vi "Theta_AxisMotorControlSetupAndHome.vi"(11 "Automation Refnum in":refnum<k7>(container)) -> (2 "Angle Serial Number":i32=40808764, 3 "Automation Refnum out":refnum<k7>)   [LabVIEW 2020]
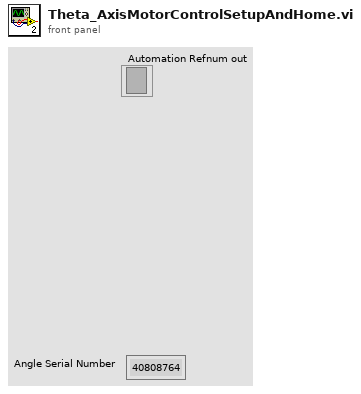
[diagram p1: front panel]
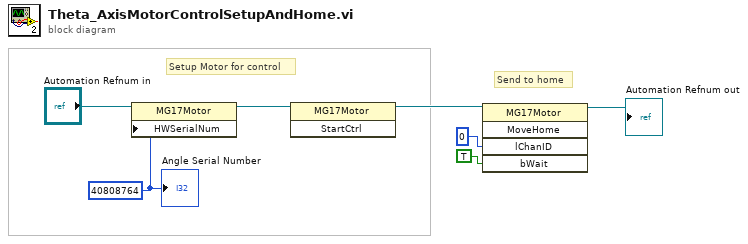
[diagram p0: block diagram]
diagram:
  w6 = 40808764 ("Serial Number Number")
  # "Setup Motor for control"
  # "Send to home"
  n1 = property on="Property Node" class="MG17Motor"(reference="Automation Refnum in", "HWSerialNum"=w6) -> (reference out=w2:refnum<k7>)  [unwired: 1 in, 1 out]
  n2 = invoke class="MG17Motor" method="StartCtrl"(reference=w2) -> (reference out=w1:refnum<k7>)  [unwired: 2 in, 2 out]
  n3 = invoke class="MG17Motor" method="MoveHome"(reference=w1, "lChanID"=0, "bWait"=TRUE) -> (reference out=→"Automation Refnum out":refnum<k7>)  [unwired: 2 in, 4 out]
  "Angle Serial Number" <- w6
